vi "Main_N5224Bv4.vi"() -> ()   [LabVIEW 2020]
uses:
  Chamber_2018/ControlCluster.ctl
  <instrlib>/Agilent PNA Series/Agilent PNA Series.lvlib
panel:
  out "Numeric 2":dbl
  out "Numeric":dbl
  in  "Tab Control":enum32{"Setup", "Results"}(tab)
  in  "File Path:":path=path "C:/Users/Lab543_Chamber/Desktop/kevin/TEST_v4.txt"
  in  "Saved by":string
  in  "File Description:":string
  out "error":errorcluster={"status"=FALSE, "code"=1073676294, "source"="VISA Read in MotorBack 2(SubVI).vi->Main_E8361C_2.vi"}
  in  "Cluster":T1={"Power Level"=-5.0, "Center Freq"=28000000000.0, "Span Freq"=2000000000.0, "Sweep Points"=5, "IF Bandwidth"=500.0, "Average Count"=1, "error"={"status"=FALSE, "code"=0, "source"=""}, "Instrument"="USB0::0x2A8D::0x2A01::MY58422353::INSTR", "Mode"=0, "Motor Range"=360, "Motor Step"=10, "VISA"="COM4"} {"Motor Step" items=["0.5 deg"=1, "1 deg"=2, "3 deg"=6, "5 deg"=10, "10 deg"=20]; "Motor Range" items=["360 deg"=360, "180 deg"=180]; "Mode" items=["Create", "Delete", "Select"]; "IF Bandwidth" format="%.3p"; "Span Freq" format="%.3p"; "Center Freq" format="%.3p"; "Power Level" format="%.2p"}
  out "Progress Bar":dbl(slide)=0.0055248618784530384 scale=0.0..1.0
  out "Gain array":dbl[][](array[numeric]) format="%#.3p"
  out "Gain Patten":dbl[][](graph)
  out "Phase array":dbl[][](array[numeric]) format="%#.3p"
  out "CurrentGain":dbl[](array[numeric])
  out "CurrentPhase":dbl[](array[numeric])
  out "Locat":dbl caption="Current Location" format="%#.1f deg."
  # "Hz"
  # "Hz"
  # "Hz"
  # "dBm"
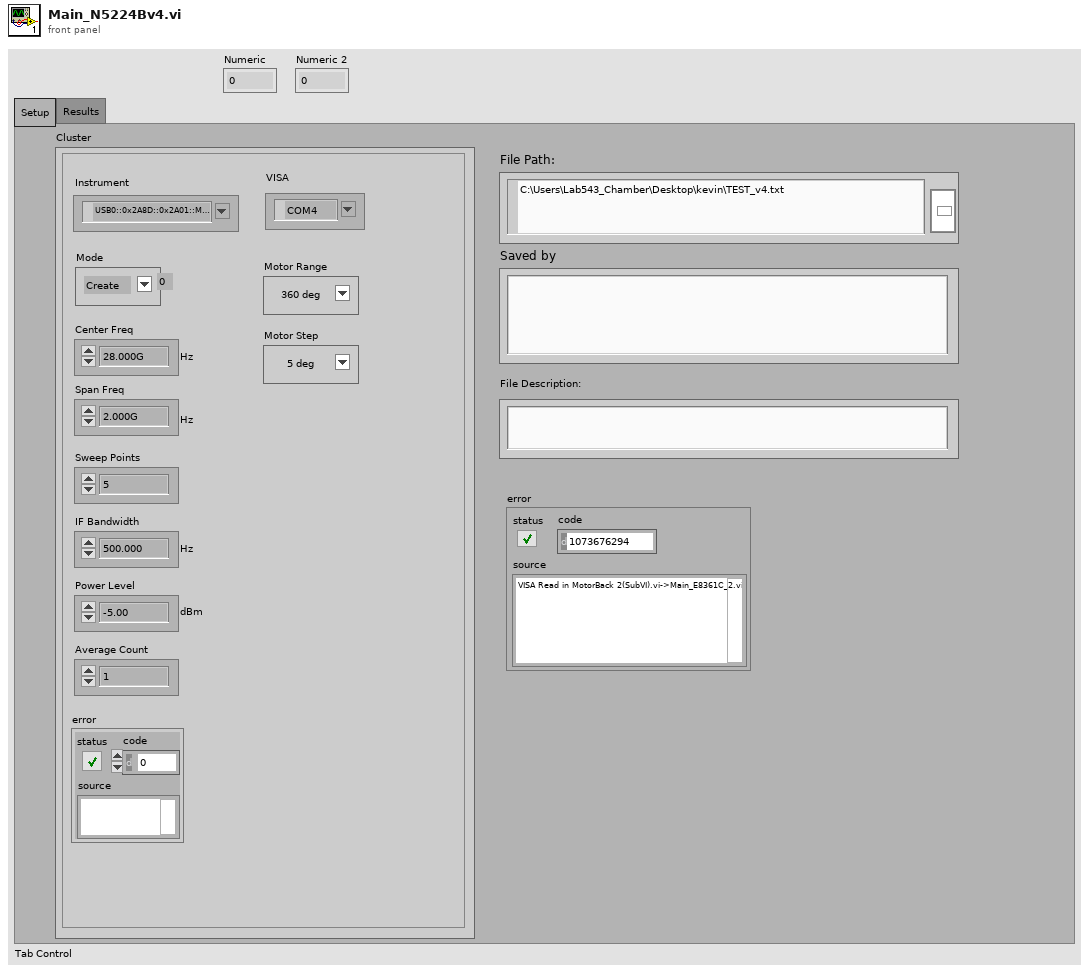
[diagram p1: front panel]
types:
  T1 = typedef "ControlCluster.ctl" = cluster{"Power Level":dbl, "Center Freq":dbl, "Span Freq":dbl, "Sweep Points":u32, "IF Bandwidth":dbl, "Average Count":i32, "error":errorcluster, "Instrument":refnum<visa-resource-name>, "Mode":u16, "Motor Range":u16, "Motor Step":u16, "VISA":refnum<visa-resource-name>}
  T2 = typedef "visaerror.ctl" = errorcluster
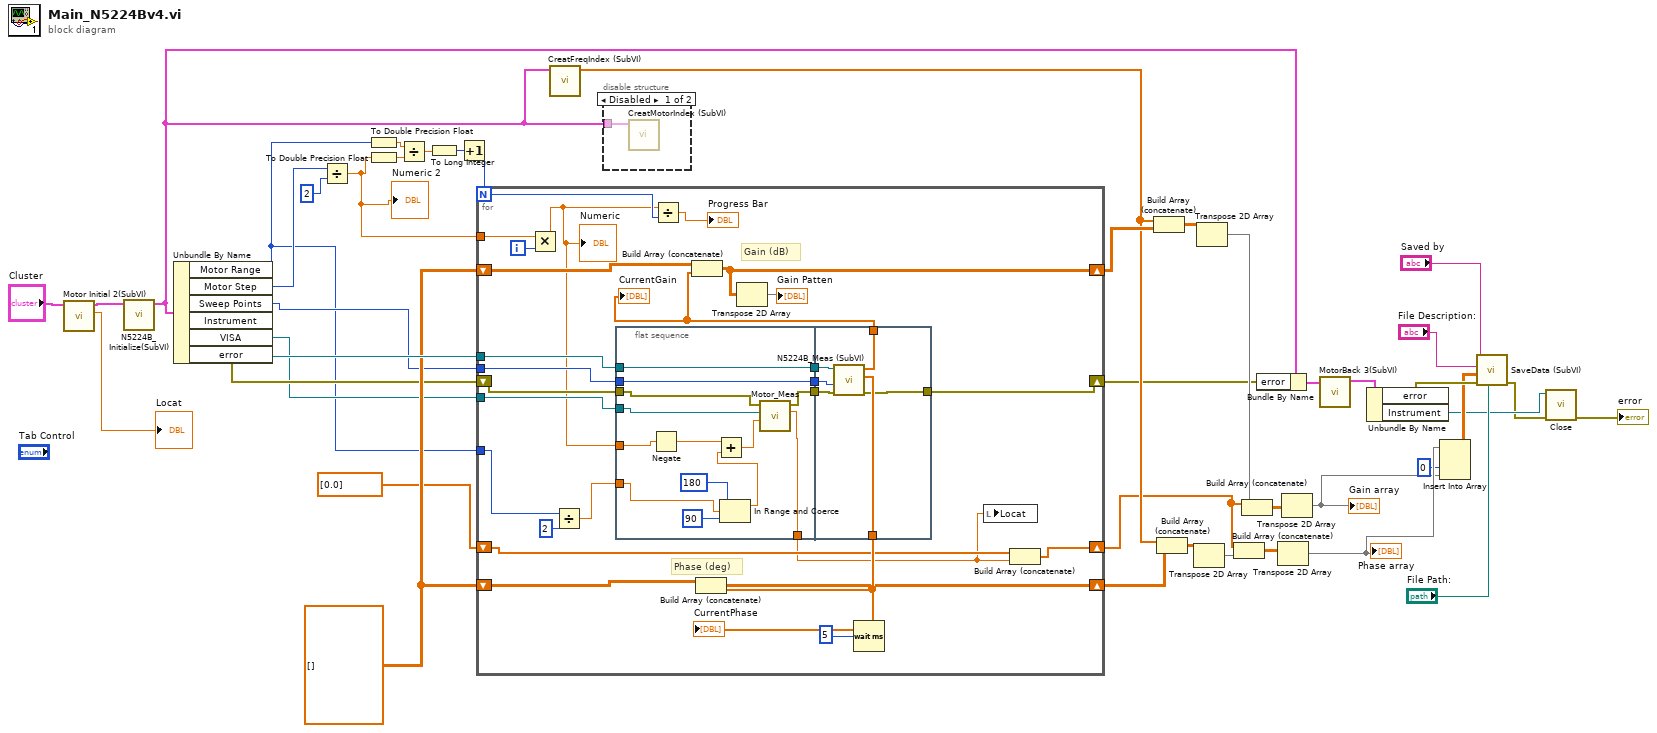
[diagram p0: block diagram]
diagram:
  w42 = dbl[][] []
  n1 = call "Motor Initial 2(SubVI).vi"("Cluster in 2"="Cluster") -> ("Locat"=→"Locat":dbl, "Cluster in 3"=w11:T1)  [unwired: 9 in]
  n2 = call "N5224B_Initialize(SubVI).vi"("Cluster in"=w11) -> ("Cluster out"=w18:T1)  [unwired: 10 in]
  n3 = Unbundle By Name(w18) -> ("Motor Range"=w4:u16, "Motor Step"=w10:u16, "Sweep Points"=w12:u32, "Instrument"=w43:refnum<visa-resource-name>, "VISA"=w8:refnum<visa-resource-name>, "error"=w9:errorcluster)
  n4 = Divide(x=w10, y=u16 2) -> (x/y=w5:dbl)
  "Numeric 2" <- w5
  n5 = To Double Precision Float(number=w4) -> (double precision float=w36:dbl)
  n6 = To Double Precision Float(number=w5) -> (double precision float=w33:dbl)
  n7 = Divide(x=w36, y=w33) -> (x/y=w34:dbl)
  n8 = To Long Integer(number=w34) -> (32bit integer=w35:i32)
  n9 = Increment(x=w35) -> (x+1=w23:i32)
  n10 = for {
    N: w23 -> [w58]
    tunnel: w43 -> [w70]
    shift-right: [w63] -> w40
    shift-left: w42 -> [w68]
    shift-right: [w66] -> w38
    shift-left: w42 -> [w65]
    shift-right: [w55] -> w7
    shift-left: w9 -> [w69]
    tunnel: w8 -> [w61]
    tunnel: w12 -> [w56]
    tunnel: w5 -> [w54]
    tunnel: w4 -> [w51]
    shift-right: [w49] -> w1
    shift-left: dbl[] [0.0] -> [w50]
    i -> [w60]
    # "Gain (dB)"
    # "Phase (deg)"
    n11 = Multiply(x=w54, y=w60) -> (x*y=w44:dbl)
    "Numeric" <- w44
    n12 = Divide(x=w51, y=2) -> (x/y=w53:dbl)
    n13 = flat-sequence {
      tunnel: w53 -> [w75]
      tunnel: w56 -> [w82]
      tunnel: w61 -> [w78]
      tunnel: w69 -> [w77]
      tunnel: w70 -> [w83]
      tunnel: [w83] -> w48
      tunnel: [w76] -> w47
      tunnel: [w82] -> w46
      tunnel: w44 -> [w73]
      tunnel: [w71] -> w45
      tunnel: [w87] -> w64
      tunnel: [w86] -> w67
      tunnel: [w85] -> w55
      tunnel: w48 -> [w89]
      tunnel: w47 -> [w88]
      tunnel: w46 -> [w84]
      frame #0 {
        n14 = Negate(x=w73) -> (-x=w74:dbl)
        n15 = In Range and Coerce(upper limit=180, x=w75, lower limit=90) -> (coerced(x)=w81:dbl)  [unwired: 1 out]
        n16 = Add(x=w74, y=w81) -> (x+y=w72:dbl)
        n17 = call "Motor_Meas.vi"("y"=w72, "COM"=w78, "error"=w77) -> ("Locat"=w71:dbl, "error 2"=w76:T2)  [unwired: 7 in]
      }
      frame #1 {
        n18 = call "N5224B_Meas (SubVI).vi"("error in (no error)"=w88, "Sample Count (401)"=w84, "VISA Refnum in"=w89) -> ("Error Out"=w85:errorcluster, "Phase"=w86:dbl[], "Gain"=w87:dbl[])  [unwired: 6 in]
      }
    }
    n19 = Divide(x=w44, y=w58) -> (x/y=→"Progress Bar":dbl)
    n20 = Build Array (concatenate)(w68, w64) -> (w63:dbl[][])
    n21 = Build Array (concatenate)(w65, w67) -> (w66:dbl[][])
    n22 = Transpose 2D Array(2D array=w63) -> (transposed array=→"Gain Patten":dbl[][])
    n23 = Wait (ms)(milliseconds to wait=u32 5) -> ()  [unwired: 1 out]
    n24 = local write "Locat"(w45) -> ()
    n25 = Build Array (concatenate)(w50, w45) -> (w49:dbl[])
    "CurrentGain" <- w64
    "CurrentPhase" <- w67
  }
  n26 = call "CreatFreqIndex (SubVI).vi"("Cluster in"=w18) -> ("FreqIndex"=w32:dbl[])  [unwired: 10 in]
  n27 = disable-structure shown="Disabled" {
    disable-tunnel: w18 -> [w90 _]
    frame Disabled {
      n28 = call "CreatMotorIndex (SubVI).vi"("Cluster in"=w90) -> ()  [unwired: 10 in, 1 out]
    }
    frame Enabled {
    }
  }
  n29 = Build Array (concatenate)(w32, w40) -> (w41:dbl[][])
  n30 = Build Array (concatenate)(w32, w38) -> (w39:dbl[][])
  n31 = Transpose 2D Array(2D array=w39) -> (transposed array=w37:dbl[][])
  n32 = Transpose 2D Array(2D array=w41) -> (transposed array=w31:dbl[][])
  n33 = Build Array (concatenate)(w1, w37) -> (w25:dbl[][])
  n34 = Build Array (concatenate)(w1, w31) -> (w24:dbl[][])
  n35 = Bundle By Name(cluster=w18, "error"=w7) -> (w6:T1)
  n36 = Transpose 2D Array(2D array=w25) -> (transposed array=w22:dbl[][])
  "Phase array" <- w22
  n37 = Transpose 2D Array(2D array=w24) -> (transposed array=w21:dbl[][])
  "Gain array" <- w21
  n38 = call "MotorBack 3(SubVI).vi"("Cluster in 2"=w6) -> ("Cluster in 3"=w26:T1)  [unwired: 10 in]
  n39 = Unbundle By Name(w26) -> ("error"=w30:errorcluster, "Instrument"=w17:refnum<visa-resource-name>)
  n40 = Insert Into Array(array=w22, index (col)=0 ("disabled index (col)"), new element=w21) -> (w20:dbl[][])  [unwired: 1 in]
  n41 = call "SaveData (SubVI).vi"("File Path:"="File Path:", "error in (no error)"=w30, "Data"=w20, "File \nDescription:"="File Description:", "Saved by"="Saved by") -> ("error out"=w16:errorcluster)  [unwired: 6 in]
  n42 = call <instrlib>:"Close.vi"("Error In (no error)"=w16, "VISA Resource Name"=w17) -> ("Error Out"=→"error":errorcluster)  [unwired: 9 in]
